vi "ClusterEscala.vi"() -> ()   [LabVIEW 2020]
panel:
  out "x*y":cluster{dbl, dbl, dbl} {"?" scale=0.0..100.0; "?" scale=0.0..100.0; "?" scale=0.0..10.0}
  in  "Cluster":T1
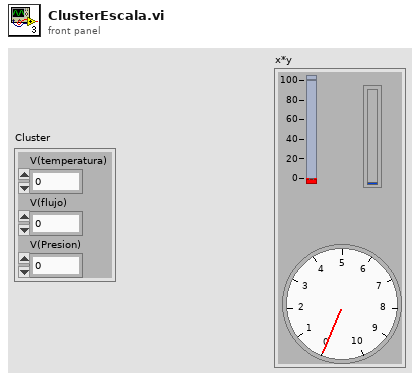
[diagram p1: front panel]
types:
  T1 = cluster{"V(temperatura)":dbl, "V(flujo)":dbl, "V(Presion)":dbl}
  T2 = cluster{"ºC/V":i32, "(l/seg)/V":i32, "(N/m^2/V)":i32}
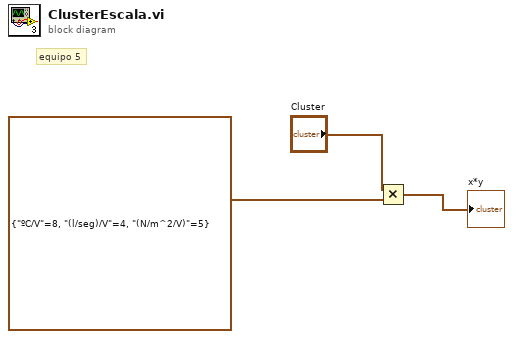
[diagram p0: block diagram]
diagram:
  # "equipo 5"
  n1 = Multiply(x="Cluster", y=T2 {"ºC/V"=8, "(l/seg)/V"=4, "(N/m^2/V)"=5}) -> (x*y=→"x*y":cluster{dbl, dbl, dbl})
